vi "Convert Date_Time.vi"(10 "Time":string="14:45:20", 11 "Date":string="06/07/13") -> (0 "error out":errorcluster, 3 "time stamp":timestamp)   [LabVIEW 2013]
doc: "Takes a string date and a string time and converts this to a timestamp."
uses:
  <vilib>/Utility/miscctls.llb/LVDateTimeRec.ctl
  <vilib>/NI/Tools/String/Tools_String.lvlib
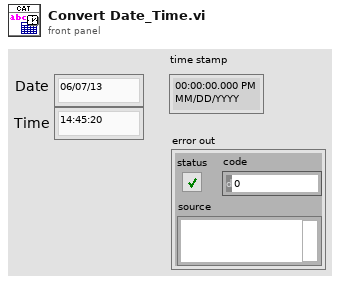
[diagram p1: front panel]
types:
  T1 = typedef "LVDateTimeRec.ctl" = cluster{"fractional second":dbl, "second":i32, "minute":i32, "hour":i32, "day of month":i32, "month":i32, "year":i32, "day of week":i32, "day of year":i32, "DST":i32}
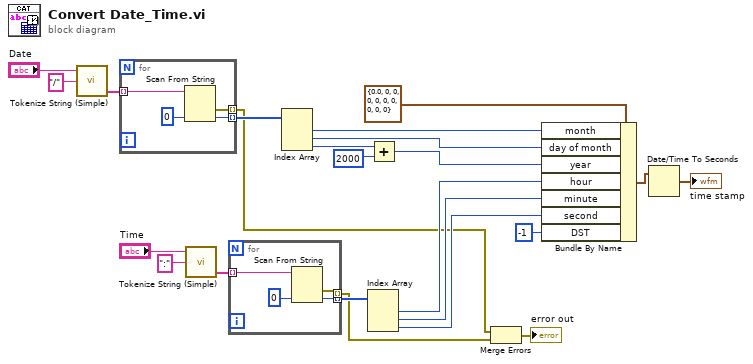
[diagram p0: block diagram]
diagram:
  n1 = call <vilib>:"Tokenize String (Simple).vi"("delimiter ([\\s\\t\\n\\r]+)"="/" ("delimiter ([\\s\\t\\n\\r]+)"), "input string"="Date") -> ("token array"=w19:string[])  [unwired: 2 in, 1 out]
  n2 = for {
    tunnel: w19 -> [w27] mode=indexing
    tunnel: [w25] -> w15 mode=indexing
    tunnel: [w24] -> w3 mode=indexing
    n3 = Scan From String(input string=w27, default 1=0 ("default value 1")) -> (error out=w24:errorcluster, output 1=w25:i32)  [unwired: 3 in, 2 out]
  }
  n4 = call <vilib>:"Tokenize String (Simple).vi"("delimiter ([\\s\\t\\n\\r]+)"=":" ("delimiter ([\\s\\t\\n\\r]+)"), "input string"="Time") -> ("token array"=w16:string[])  [unwired: 2 in, 1 out]
  n5 = for {
    tunnel: w16 -> [w31] mode=indexing
    tunnel: [w29] -> w11 mode=indexing
    tunnel: [w28] -> w4 mode=indexing
    n6 = Scan From String(input string=w31, default 1=0 ("default value 1")) -> (error out=w28:errorcluster, output 1=w29:i32)  [unwired: 3 in, 2 out]
  }
  n7 = Index Array(array=w15) -> (element #1=w14:i32, element #2=w13:i32, element #3=w7:i32)  [unwired: 3 in]
  n8 = Index Array(array=w11) -> (element #1=w10:i32, element #2=w9:i32, element #3=w8:i32)  [unwired: 3 in]
  n9 = Add(x=w7, y=2000) -> (x+y=w5:i32)
  n10 = Merge Errors(w3, w4) -> (→"error out":errorcluster)
  n11 = Bundle By Name(cluster=T1 {"fractional second"=0.0, "second"=0, "minute"=0, "hour"=0, "day of month"=0, "month"=0, "year"=0, "day of week"=0, "day of year"=0, "DST"=0} ("date time rec"), "month"=w14, "day of month"=w13, "year"=w5, "hour"=w10, "minute"=w9, "second"=w8, "DST"=-1) -> (w20:T1)
  n12 = Date/Time To Seconds(2:w20) -> (0:→"time stamp":timestamp)  [unwired: 1 in]
